vi "7.1.vi"() -> ()   [LabVIEW 2017]
uses:
  <vilib>/measure/NI_MABase.lvlib
panel:
  out "XY Graph":cluster{"Y":dbl[], "Y":dbl[]}(graph)
  in  "amplitude 2":dbl=1.0 caption="幅值" format="%0.2p"
  in  "frequency 2":dbl=10.0 caption="频率" format="%0.2p"
  in  "phase 2":dbl caption="相位" format="%.2p"
  in  "amplitude":dbl=1.0 caption="幅值" format="%0.2p"
  in  "frequency":dbl=10.0 caption="频率" format="%0.2p"
  in  "phase":dbl caption="相位" format="%.2p"
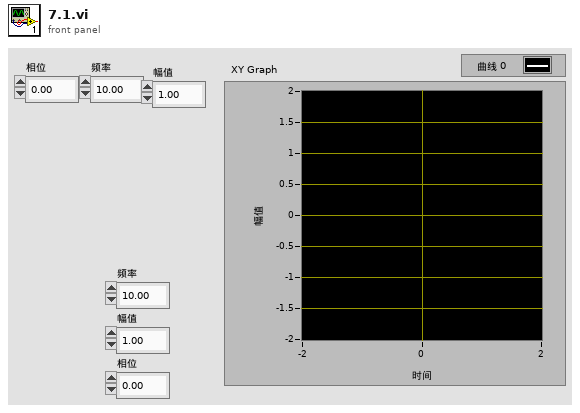
[diagram p1: front panel]
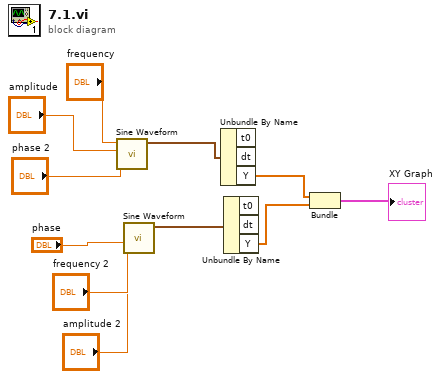
[diagram p0: block diagram]
diagram:
  n1 = call <vilib>:"Sine Waveform.vi"("phase"="phase 2", "amplitude"="amplitude", "frequency"="frequency") -> ("signal out"=w11:waveform(dbl))  [unwired: 7 in, 1 out]
  n2 = call <vilib>:"Sine Waveform.vi"("phase"="phase", "amplitude"="amplitude 2", "frequency"="frequency 2") -> ("signal out"=w9:waveform(dbl))  [unwired: 7 in, 1 out]
  n3 = Unbundle By Name(w11) -> ("Y"=w8:dbl[])  [unwired: 2 out]
  n4 = Unbundle By Name(w9) -> ("Y"=w7:dbl[])  [unwired: 2 out]
  n5 = Bundle("Y"=w8, "Y"=w7) -> (→"XY Graph":cluster{"Y":dbl[], "Y":dbl[]})  [unwired: 1 in]
